vi "DAQmx Timing (Handshaking).vi"(0 "task/channels in":refnum<k21>, 1 "sample mode":i32(ring)=10178 items=["Finite Samples"=10178, "Continuous Samples"=10123, "Hardware Timed Single Point"=12522], 2 "samples per channel":i32=1000, 11 "error in":errorcluster) -> (4 "task out":refnum<k21>, 15 "error out":errorcluster)   [LabVIEW 2011]
doc: "Determines the number of digital samples to acquire or generate using digital handshaking between the device and a peripheral device."
uses:
  C:/Program Files/National Instruments/LabVIEW 2011/resource/objmgr/daqmx.rc
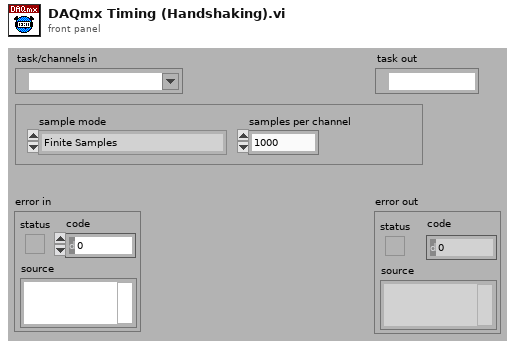
[diagram p1: front panel]
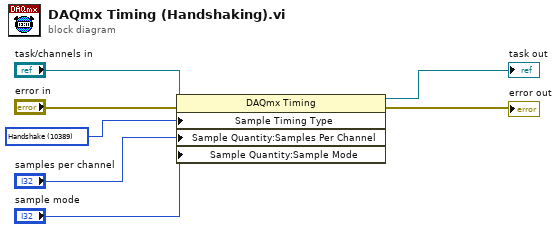
[diagram p0: block diagram]
diagram:
  w1 = 10389 items=["Sample Clock"=10388, "Handshake"=10389, "Implicit"=10451, "On Demand"=10390, "Change Detection"=12504] ("Sample Timing Type")
  n1 = property class="DAQmx Timing"(reference="task/channels in", error in="error in", "Sample Timing Type"=w1, "Sample Quantity:Samples Per Channel"="samples per channel", "Sample Quantity:Sample Mode"="sample mode") -> (reference out=→"task out":refnum<k21>, error out=→"error out":errorcluster)
